vi "labHolo_path.vi"(2 "sub folder or file (path)  [ignored if str is not empty]":path, 3 "sub folder or file (str)":string) -> (0 "Exists?":bool, 1 "labHolo path":path)   [LabVIEW 2023]
panel:
  out "sub folder names 2":string[](array[string])
  out "sub filenames 2":string[](array[string])
  out "sub folder names":string[](array[string])
  out "sub filenames":string[](array[string])
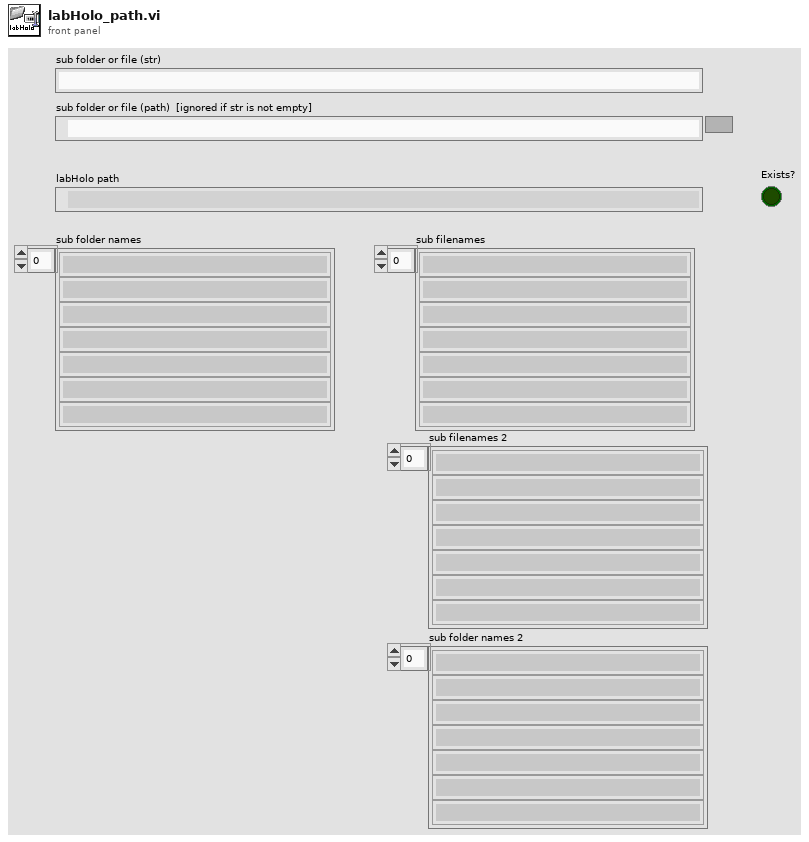
[diagram p1: front panel]
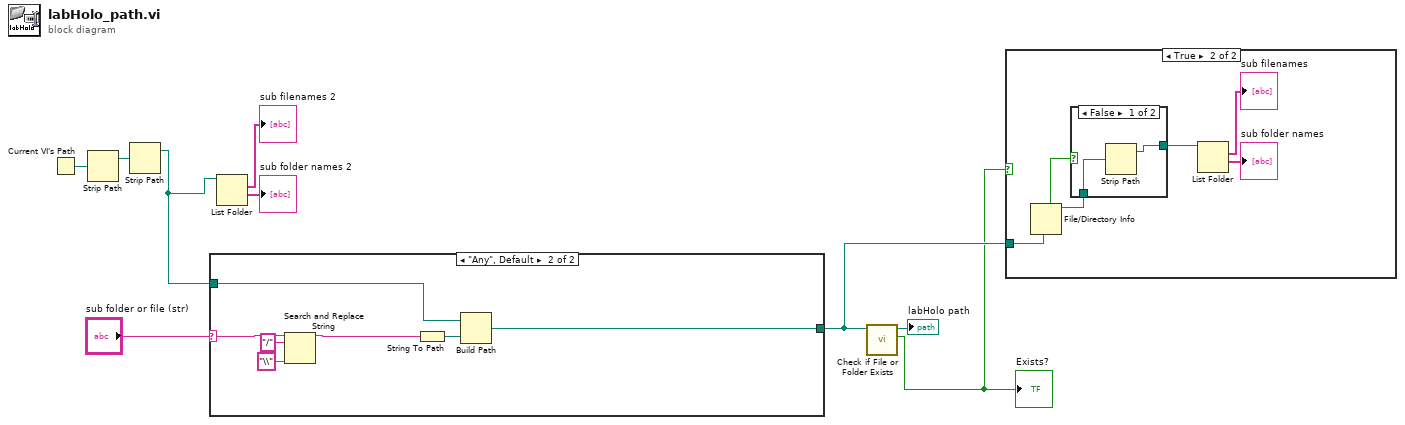
[diagram p0: block diagram]
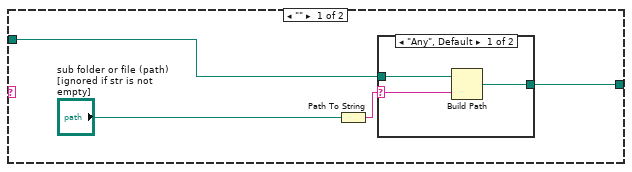
[diagram p4: hidden frame]
diagram:
  n1 = Current VI's Path() -> (path=w9:path)
  n2 = Strip Path(path=w9) -> (stripped path=w8:path)  [unwired: 1 out]
  n3 = Strip Path(path=w8) -> (stripped path=w2:path)  [unwired: 1 out]
  n4 = case shown="\"Any\", Default" "sub folder or file (str)" {
    selector: "sub folder or file (str)" -> [_ w21]
    tunnel: w2 -> [w13 w23]
    tunnel: [w10 w24] -> w5
    frame "" {
      n5 = Path To String(path="sub folder or file (path)  [ignored if str is not empty]") -> (string=w11:string)
      n6 = case shown="\"Any\", Default" w11 {
        selector: w11 -> [w16 _]
        tunnel: w13 -> [w15 w17]
        tunnel: [w14 w17] -> w10
        frame "Any", Default {
          n7 = Build Path(base path=w15, name or relative path=w16) -> (appended path=w14:path)
        }
        frame "" {
        }
      }
    }
    frame "Any", Default {
      n8 = Search and Replace String(input string=w21, search string="/", replace string="\\" ("replace string (\"\")")) -> (result string=w20:string)  [unwired: 5 in, 3 out]
      n9 = String To Path(string=w20) -> (path=w22:path)
      n10 = Build Path(base path=w23, name or relative path=w22) -> (appended path=w24:path)
    }
  }
  n11 = List Folder(path=w2) -> (filenames=→"sub filenames 2":string[], folder names=→"sub folder names 2":string[])  [unwired: 3 in, 2 out]
  n12 = call <vilib>:"Check if File or Folder Exists.vi"("path"=w5) -> ("file or folder exists?"=w1:bool, "dup path"=→"labHolo path":path)  [unwired: 8 in, 1 out]
  "Exists?" <- w1
  n13 = case shown="True" w1 {
    tunnel: w5 -> [_ w28]
    frame False {
    }
    frame True {
      n14 = File/Directory Info(path=w28) -> (path out=w25:path, directory=w27:bool)  [unwired: 1 in, 5 out]
      n15 = case shown="False" w27 {
        tunnel: [w32 w33] -> w26
        tunnel: w25 -> [w31 w33]
        frame False {
          n16 = Strip Path(path=w31) -> (stripped path=w32:path)  [unwired: 1 out]
        }
        frame True {
        }
      }
      n17 = List Folder(path=w26) -> (filenames=→"sub filenames":string[], folder names=→"sub folder names":string[])  [unwired: 3 in, 2 out]
    }
  }
